vi "ReadConfigFiles.vi"(4 "Variable":string[](array[string])=["Center"], 6 "Control":string[](array[string])=["Center Voltage"], 8 "error in":errorcluster, 9 "Pages":refnum<vi>[](array[refnum]), 10 "reference":refnum<vi>, 11 "variant in":variant) -> (0 "error out":errorcluster, 3 "variant out":variant)   [LabVIEW 2013]
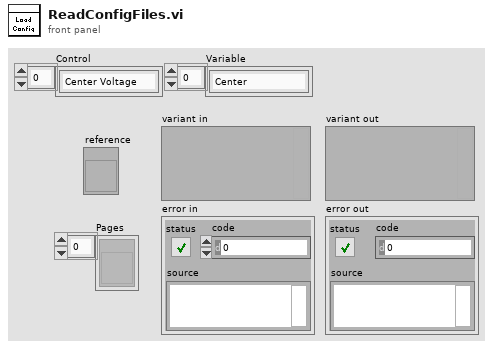
[diagram p1: front panel]
types:
  T1 = enum16{"open", "replace", "create", "open or create", "replace or create", "replace or create with confirmation"}
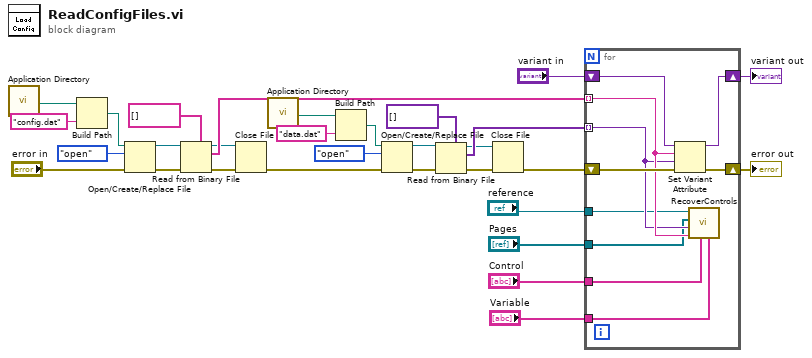
[diagram p0: block diagram]
diagram:
  n1 = call <vilib>:"Application Directory.vi"() -> ("Application Directory"=w7:path)
  n2 = Build Path(base path=w7, name or relative path="config.dat") -> (appended path=w9:path)
  n3 = Open/Create/Replace File(file path (use dialog)=w9, error in="error in", operation (0:open)=T1."open") -> (refnum out=w17:refnum<file>, error out=w18:errorcluster)  [unwired: 3 in, 1 out]
  n4 = Read from Binary File(5:string[] [] ("names"), 8:w18, 11:w17) -> (0:w15:errorcluster, 2:w25:string[], 3:w16:refnum<file>)  [unwired: 3 in, 1 out]
  n5 = Close File(refnum=w16, error in=w15) -> (error out=w27:errorcluster)  [unwired: 1 out]
  n6 = call <vilib>:"Application Directory.vi"() -> ("Application Directory"=w14:path)
  n7 = Build Path(base path=w14, name or relative path="data.dat") -> (appended path=w12:path)
  n8 = Open/Create/Replace File(file path (use dialog)=w12, error in=w27, operation (0:open)=T1."open") -> (refnum out=w20:refnum<file>, error out=w19:errorcluster)  [unwired: 3 in, 1 out]
  n9 = Read from Binary File(5:variant[] [] ("values"), 8:w19, 11:w20) -> (0:w22:errorcluster, 2:w26:variant[], 3:w21:refnum<file>)  [unwired: 3 in, 1 out]
  n10 = Close File(refnum=w21, error in=w22) -> (error out=w28:errorcluster)  [unwired: 1 out]
  n11 = for {
    tunnel: w25 -> [w36] mode=indexing
    tunnel: w26 -> [w35] mode=indexing
    shift-right: [w39] -> w6
    shift-left: "variant in" -> [w40]
    shift-right: [w38] -> w5
    shift-left: w28 -> [w37]
    tunnel: "reference" -> [w34]
    tunnel: "Pages" -> [w33]
    tunnel: "Control" -> [w32]
    tunnel: "Variable" -> [w31]
    n12 = Set Variant Attribute(Variant=w40, name=w36, value=w35, error in=w37) -> (Variant out=w39:variant, error out=w38:errorcluster)  [unwired: 1 out]
    n13 = call "RecoverControls.vi"("Variable"=w31, "Control"=w32, "Name"=w36, "Value"=w35, "Pages"=w33, "reference"=w34) -> ()  [unwired: 6 in]
  }
  "variant out" <- w6
  "error out" <- w5
